vi "LSC218 status FGV.vi"(3 "Action":T4, 5 "LSC218 status in":T3) -> (2 "LSC218 statuses":T2(array[cluster]))   [LabVIEW 2017, in "Magnet module.lvlib"]
uses:
  ctl/FGV action.ctl
  ctl/TM Revision.ctl
  Magnet module.lvlib
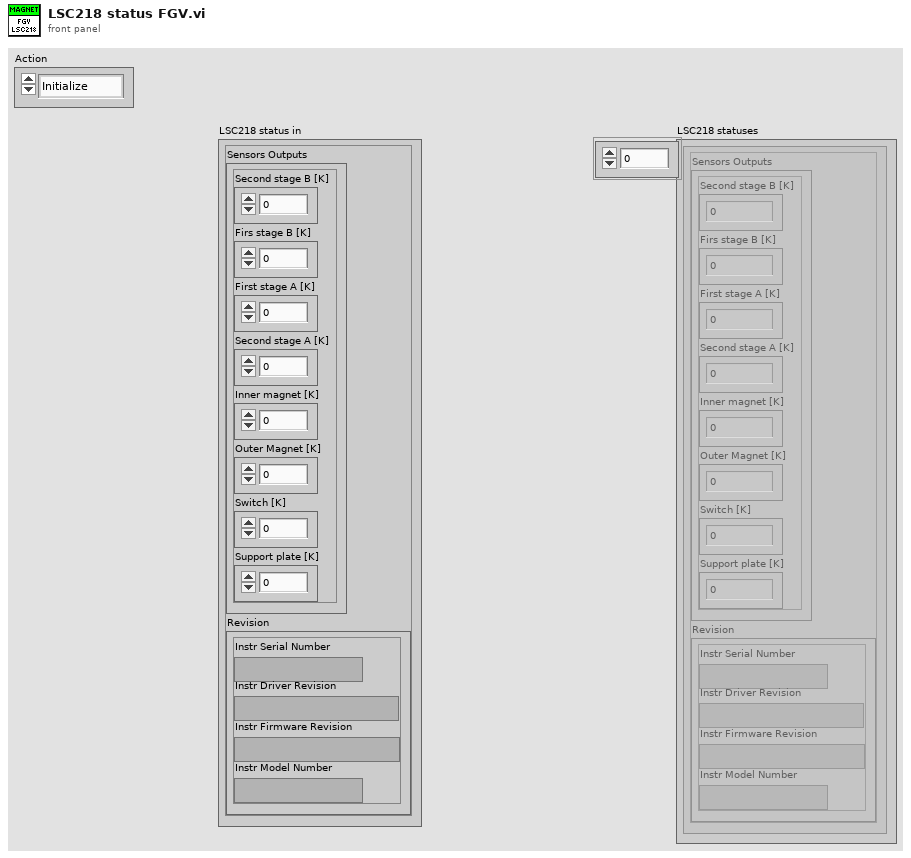
[diagram p1: front panel]
types:
  T1 = typedef "Magnet module.lvlib/TM Revision.ctl" = cluster{"Instr Serial Number":string, "Instr Driver Revision":string, "Instr Firmware Revision":string, "Instr Model Number":string}
  T2 = cluster{"Sensors Outputs":cluster{"Second stage B [K]":dbl, "Firs stage B [K]":dbl, "First stage A [K]":dbl, "Second stage A [K]":dbl, "Inner magnet [K]":dbl, "Outer Magnet [K]":dbl, "Switch [K]":dbl, "Support plate [K]":dbl}, "Revision":T1}[]
  T3 = cluster{"Sensors Outputs":cluster{"Second stage B [K]":dbl, "Firs stage B [K]":dbl, "First stage A [K]":dbl, "Second stage A [K]":dbl, "Inner magnet [K]":dbl, "Outer Magnet [K]":dbl, "Switch [K]":dbl, "Support plate [K]":dbl}, "Revision":T1}
  T4 = typedef "Magnet module.lvlib/FGV action.ctl" = enum16{"Initialize", "Update", "Read", "Action"}
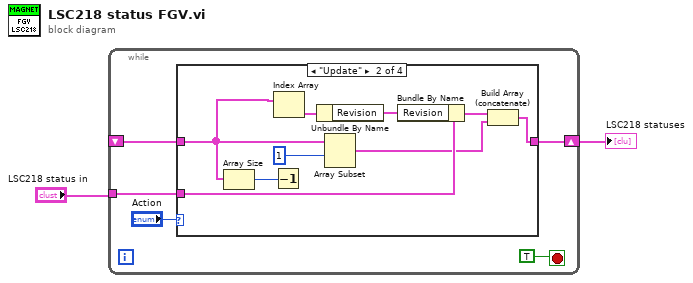
[diagram p0: block diagram]
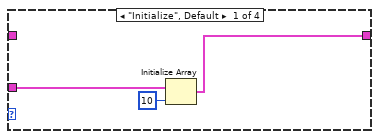
[diagram p2: hidden frame]
diagram:
  n1 = while {
    shift-right: [w6] -> w1
    shift-left: _ -> [w3]
    tunnel: "LSC218 status in" -> [w4]
    stop <- TRUE stop-if-true
    n2 = case shown="\"Update\"" "Action" {
      tunnel: w3 -> [_ w12 w20 w21]
      tunnel: [w8 w11 w20 w21] -> w6
      tunnel: w4 -> [w9 w19 _ _]
      frame "Initialize", Default {
        n3 = Initialize Array(w9, 10 ("dimension size")) -> (w8:T2)
      }
      frame "Update" {
        n4 = Array Size(array=w12) -> (size(s)=w13:i32)
        n5 = Decrement(x=w13) -> ()  [unwired: 1 out]
        n6 = Index Array(array=w12) -> (element=w16:T3)  [unwired: 1 in]
        n7 = Unbundle By Name(w16) -> ("Revision"=w18:T1)
        n8 = Array Subset(array=w12, index=1) -> (w14:T2)  [unwired: 1 in]
        n9 = Bundle By Name(cluster=w19, "Revision"=w18) -> (w15:T3)
        n10 = Build Array (concatenate)(w15, w14) -> (w11:T2)
      }
      frame "Read" {
      }
      frame "Action" {
      }
    }
  }
  "LSC218 statuses" <- w1
